vi "petri Tracking.vi"() -> ()   [LabVIEW 2016]
uses:
  <vilib>/vision/driver/NI_Vision_Acquisition_Software.lvlib
  <vilib>/userdefined/High Color/IMAQdx.ctl
panel:
  out "Numeric":i32
  out "Positions XY":dbl[][](array[numeric])=[[100.0, 200.0], [300.0, 700.0], [500.0, 600.0], [700.0, 1500.0], [900.0, 1500.0]]
  out "error out":errorcluster
  in  "next":bool
  in  "petri run":bool
  out "Image Out":T1(plugin-control)
  out "Cells parameters":string[][](table)
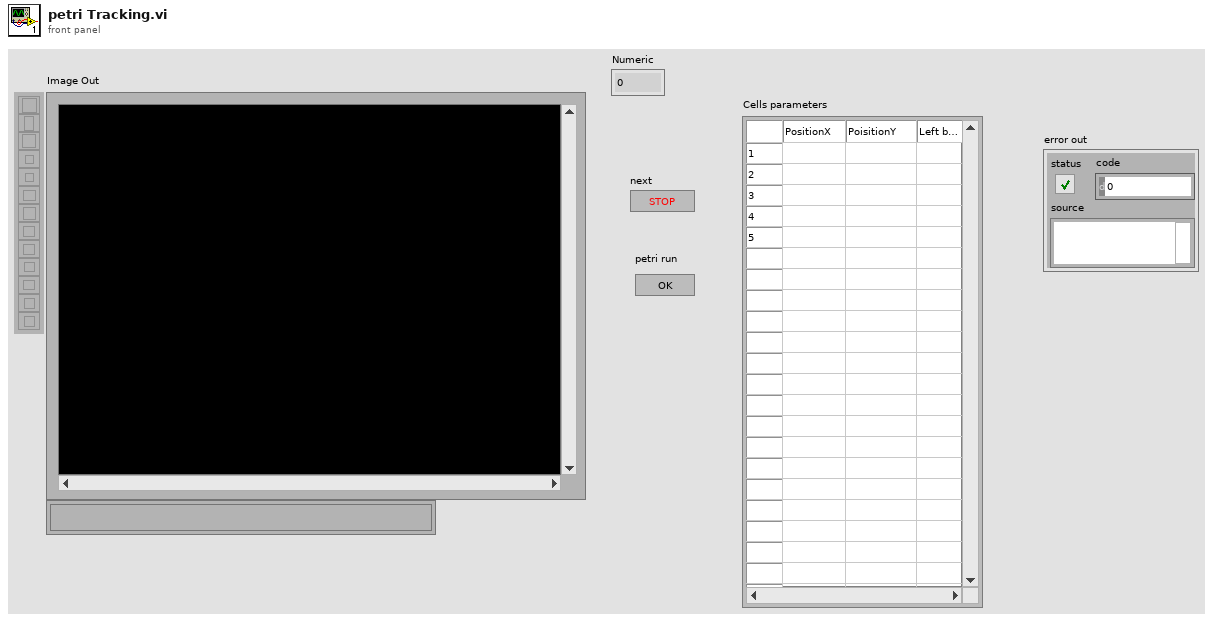
[diagram p1: front panel]
types:
  T1 = typedef "IMAQ Image.ctl" = refnum<image>
  T2 = typedef "IMAQdx.ctl" = refnum<k21>
  T3 = cluster{"Name":string, "Type":enum16{"Line", "Broken Line", "Free Hand Line", "Rotated Rectangle", "Oval", "Polygon", "Free Hand", "Bitmap", "Text"}, "Coordinates":i32[], "Colors":u32[], "Drawing Mode":u32, "Text":string, "Results":cluster{"Process ID":string, "Measure":u16, "Name":string, "String Format":u16, "Width":i16, "Precision":i16, "True String":string, "False String":string}[], "Font, Size & Style":cluster{"Desired Font (Application)":enum16{"User-specified Font", "Application Font", "System Font", "Dialog Font"}, "[User-specified Font]":cluster{"Font Name":string, "Size":i16, "Strikeout?":bool, "Italic?":bool, "Underline?":bool, "Outline?":bool, "Shadow?":bool, "Bold?":bool, "Rotation Angle":dbl}, "Horizontal Alignment":i16, "Vertical Alignment":i16}, "Image File Path":path, "Use Keying Color":bool}[]
  T4 = cluster{"Left":i32, "Top":i32, "Right":i32, "Bottom":i32}
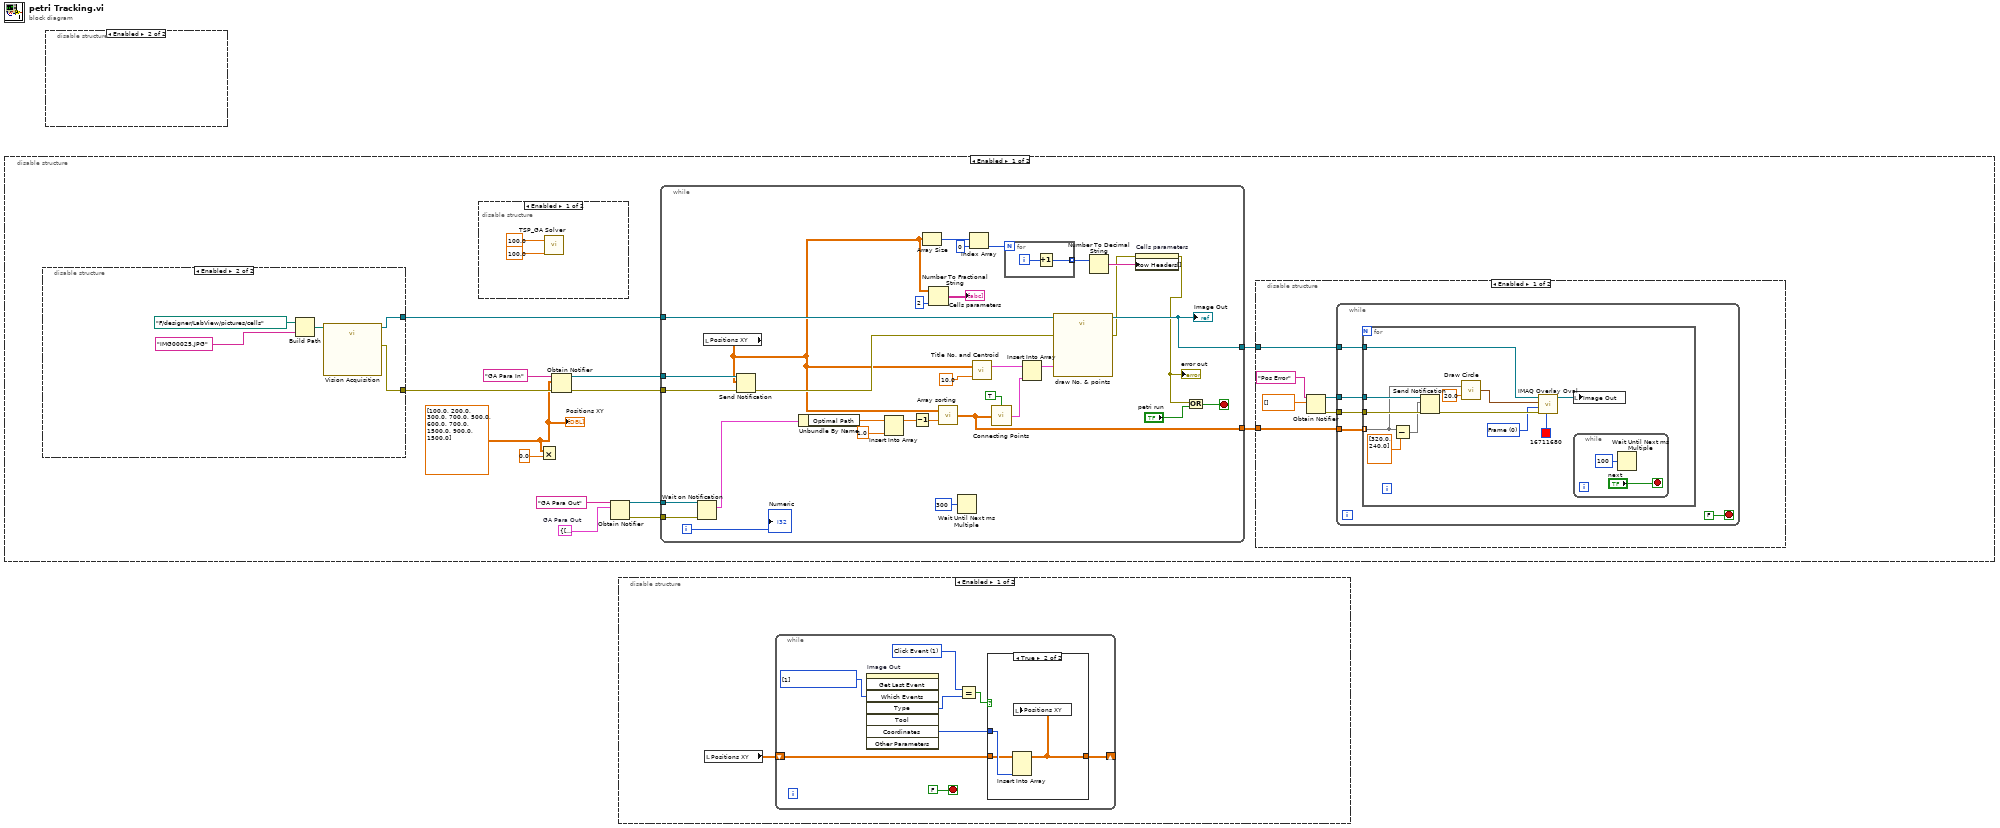
[diagram p0: block diagram]
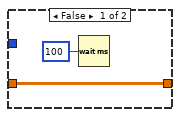
[diagram p2: hidden frame]
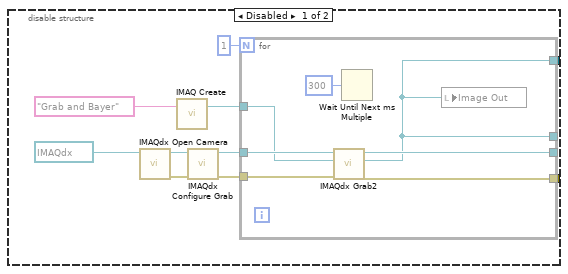
[diagram p5: hidden frame]
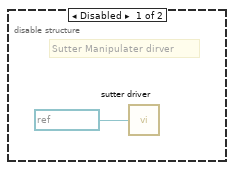
[diagram p8: hidden frame]
diagram:
  n1 = disable-structure shown="Enabled" {
    frame Enabled {
      w9 = cluster{"Optimal Path":dbl[], "Total Dist":dbl} {"Optimal Path"=[], "Total Dist"=0.0}  # GA Para Out
      w2 = dbl[][] [[100.0, 200.0], [300.0, 700.0], [500.0, 600.0], [700.0, 1500.0], [900.0, 1500.0]] ("Positions XY")
      n2 = disable-structure shown="Enabled" {
        disable-tunnel: [w25 w33] -> w12
        disable-tunnel: [w24 w34] -> w11
        frame Disabled {
          n3 = call <vilib>:"IMAQdx Open Camera.vi"("Session In"=T2 "cam1") -> ("error out"=w19:errorcluster, "Session Out"=w20:T2)  [unwired: 2 in, 7 out]
          n4 = call "IMAQ Create"("Image Name"="Grab and Bayer") -> ("New Image"=w17:T1)  [unwired: 3 in, 2 out]
          n5 = call <vilib>:"IMAQdx Configure Grab.vi"("error in"=w19, "Session In"=w20) -> ("error out"=w22:errorcluster, "Session Out"=w21:T2)  [unwired: 8 out]
          n6 = for {
            N: 1 -> [_]
            tunnel: w17 -> [w30]
            tunnel: w22 -> [w31]
            tunnel: w21 -> [w32]
            tunnel: [w29] -> _
            tunnel: [w28] -> w25
            tunnel: [w26] -> _
            tunnel: [w26] -> w24
            n7 = call <vilib>:"IMAQdx Grab2.vi"("error in"=w31, "Image In"=w30, "Session In"=w32) -> ("error out"=w28:errorcluster, "Image Out"=w26:T1, "Session Out"=w29:T2)  [unwired: 5 in, 1 out]
            n8 = Wait Until Next ms Multiple(millisecond multiple=u32 300) -> ()  [unwired: 1 out]
            n9 = local write "Image Out"(w26) -> ()
          }
        }
        frame Enabled {
          n10 = Build Path(base path=path "F:/designer/LabView/pictures/cells" ("file path (dialog if empty)"), name or relative path="IMG00025.JPG" ("名称或相对路径")) -> (appended path=w36:path)
          n11 = call "Vision Acquisition"("Image Path"=w36) -> ("Image Out"=w34:T1, "error out"=w33:errorcluster)  [unwired: 25 in]
        }
      }
      n12 = disable-structure shown="Enabled" {
        frame Enabled {
          n13 = call "TSP_GA Solver.vi"("pop_size"=100.0, "Number of Iterative"=100.0) -> ()  [unwired: 1 in]
        }
        frame Disabled {
        }
      }
      n14 = Multiply(x=w2, y=0.0 ("Numeric")) -> ()  [unwired: 1 out]
      n15 = Obtain Notifier(name (unnamed)="GA Para In", notification data type=w2, error in (no error)=w12) -> (notifier out=w4:refnum<notifier>, error out=w3:errorcluster)  [unwired: 1 in, 1 out]
      n16 = Obtain Notifier(name (unnamed)="GA Para Out", notification data type=w9) -> (notifier out=w8:refnum<notifier>, error out=w7:errorcluster)  [unwired: 2 in, 1 out]
      n17 = while {
        tunnel: w4 -> [w65]
        tunnel: w3 -> [w67]
        tunnel: w11 -> [w78]
        tunnel: [w77] -> w5
        tunnel: [w76] -> w6
        tunnel: w8 -> [w71]
        tunnel: w7 -> [w70]
        i -> [w63]
        stop <- w75 stop-if-true
        n18 = Wait on Notification(notifier=w71, error in (no error)=w70) -> (notification=w69:cluster{"Optimal Path":dbl[], "Total Dist":dbl})  [unwired: 2 in, 3 out]
        n19 = local read "Positions XY"() -> (w64:dbl[][])
        n20 = Send Notification(notification=w64, notifier=w65, error in (no error)=w67) -> (error out=w66:errorcluster)  [unwired: 1 out]
        n21 = Unbundle By Name(w69) -> ("Optimal Path"=w68:dbl[])
        n22 = Insert Into Array(array=w68, new element=1.0 ("element")) -> (w81:dbl[])  [unwired: 1 in]
        n23 = Decrement(x=w81) -> (x-1=w83:dbl[])
        n24 = Array Size(array=w64) -> (size(s)=w91:i32[])
        n25 = Number To Fractional String(number=w64, precision (6)=i16 2 ("精度(6)")) -> (F-format string=→"Cells parameters":string[][])  [unwired: 2 in]
        n26 = call "Array sorting.vi"("index"=w83, "Array In"=w64) -> ("Array Out"=w77:dbl[][])
        n27 = Wait Until Next ms Multiple(millisecond multiple=u32 300) -> ()  [unwired: 1 out]
        n28 = Index Array(array=w91, index=0 ("索引")) -> (element=w89:i32)
        n29 = call "Title No. and Centroid.vi"("半径"=10.0, "Particle Measurements (Pixels)"=w64) -> ("输出数组"=w86:T3)  [unwired: 1 out]
        n30 = call "Connecting Points.vi"("Boolean"=TRUE, "数组"=w77) -> ("输出数组"=w84:T3)  [unwired: 2 in]
        n31 = for {
          N: w89 -> [_]
          tunnel: [w95] -> w88 mode=indexing
          i -> [w96]
          n32 = Increment(x=w96) -> (x+1=w95:i32)
        }
        n33 = Insert Into Array(array=w86, new element=w84) -> (w85:T3)  [unwired: 1 in]
        n34 = call "draw No. & points"("Image In"=w78, "Parameters (Overlay 1)"=w85, "error in"=w66) -> ("Image Out"=w76:T1, "error out"=w73:errorcluster)  [unwired: 23 in]
        "Image Out" <- w76
        n35 = Number To Decimal String(number=w88) -> (decimal integer string=w87:string[])  [unwired: 1 in]
        n36 = property on="Cells parameters" class="Tbl (strict)"(error in=w73, "Row Headers[]"=w87) -> (error out=w72:errorcluster)  [unwired: 1 in, 1 out]
        "error out" <- w72
        n37 = Or(x=w72, y="petri run") -> (x .or. y?=w75:bool)
        "Numeric" <- w63
      }
      n38 = disable-structure shown="Enabled" {
        disable-tunnel: w6 -> [w39 _]
        disable-tunnel: w5 -> [w38 _]
        frame Enabled {
          n39 = Obtain Notifier(name (unnamed)="Pos Error", notification data type=dbl[] []) -> (notifier out=w41:refnum<notifier>, error out=w40:errorcluster)  [unwired: 2 in, 1 out]
          n40 = while {
            tunnel: w38 -> [w48]
            tunnel: w41 -> [w47]
            tunnel: w40 -> [w46]
            tunnel: w39 -> [w45]
            stop <- FALSE stop-if-true
            n41 = for {
              tunnel: w48 -> [w54] mode=indexing
              tunnel: w47 -> [w60]
              tunnel: w46 -> [w59]
              tunnel: w45 -> [w56]
              w51 = u32 0 items=["Frame", "Fill"] ("Drawing Mode (Frame)")
              n42 = Subtract(x=w54, y=dbl[] [320.0, 240.0]) -> (x-y=w57:dbl[])
              n43 = Send Notification(notification=w57, notifier=w60, error in (no error)=w59) -> (error out=w55:errorcluster)  [unwired: 1 out]
              n44 = call "Draw Circle.vi"("radius"=20.0, "Pos XY"=w54) -> ("Bound out"=w52:T4)
              n45 = call "IMAQ Overlay Oval"("Color"=u32 16711680, "error in (no error)"=w55, "Drawing Mode (Frame)"=w51, "Bounding Rectangle"=w52, "Image"=w56) -> ("Image Out"=w49:T1)  [unwired: 5 in, 1 out]
              n46 = local write "Image Out"(w49) -> ()
              n47 = while {
                stop <- "next" stop-if-true
                n48 = Wait Until Next ms Multiple(millisecond multiple=u32 100) -> ()  [unwired: 1 out]
              }
            }
          }
        }
        frame Disabled {
        }
      }
      "Positions XY" <- w2
    }
    frame Disabled {
    }
  }
  n49 = disable-structure shown="Enabled" {
    frame Disabled {
      # "Sutter Manipulater dirver"
      n50 = call "sutter driver.vi"("VISA resource name"=refnum<visa-resource-name> "COM1") -> ()
    }
    frame Enabled {
    }
  }
  n51 = disable-structure shown="Enabled" {
    frame Enabled {
      n52 = local read "Positions XY"() -> (w98:dbl[][])
      n53 = while {
        shift-right: [w101] -> _
        shift-left: w98 -> [w102]
        stop <- FALSE stop-if-true
        w100 = 1 items=["No Event"=0, "Click Event"=1, "Draw Event"=2, "Size Event"=4, "Scroll Event"=5, "Double Click Event"=8]
        w99 = i32[] [1] items=["No Event"=0, "Click Event"=1, "Draw Event"=2, "Size Event"=4, "Scroll Event"=5, "Double Click Event"=8] ("Which Events")
        n54 = invoke on="Image Out" class="ImageControl" method="Get Last Event"("Which Events"=w99) -> ("Type"=w105:i32, "Coordinates"=w106:i32[])  [unwired: 7 in, 6 out]
        n55 = Equal?(x=w100, y=w105) -> (x = y?=w103:bool)
        n56 = case shown="True" w103 {
          tunnel: w106 -> [_ w111]
          tunnel: w102 -> [w107 w110]
          tunnel: [w107 w109] -> w101
          frame False {
            n57 = Wait (ms)(milliseconds to wait=u32 100 ("等待时间（毫秒）")) -> ()  [unwired: 1 out]
          }
          frame True {
            n58 = Insert Into Array(array=w110, new element=w111) -> (w109:dbl[][])  [unwired: 2 in]
            n59 = local write "Positions XY"(w109) -> ()
          }
        }
      }
    }
    frame Disabled {
    }
  }
